vi "INTEGER_BHBL.vi"(0 "int16":i16) -> (1 "Lvalue":u8 format="%x", 2 "HValue":u8 format="%x")   [LabVIEW 2011]
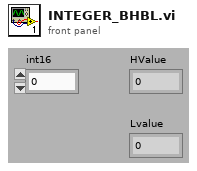
[diagram p1: front panel]
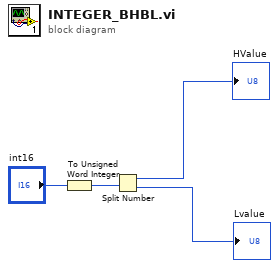
[diagram p0: block diagram]
diagram:
  n1 = To Unsigned Word Integer(number="int16") -> (unsigned 16bit integer=w4:u16)
  n2 = Split Number(x=w4) -> (hi(x)=→"HValue":u8, lo(x)=→"Lvalue":u8)
